vi "testInvalidApplicationRefnum.vi"() -> ()   [LabVIEW 2019, in "AssertionTest.lvlib" / "AssertNotRefnum.lvlib"]
uses:
  AssertNotRefnum.lvlib
  Assertion/Assertion.lvlib
panel:
  out "error out":errorcluster
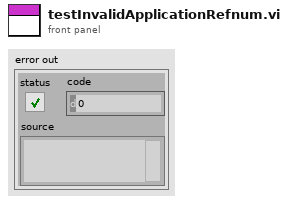
[diagram p1: front panel]
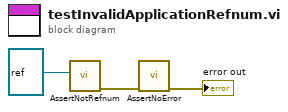
[diagram p0: block diagram]
diagram:
  n1 = call "AssertNotRefnum.vi"("Refnum"=refnum<vi> refnum ("App Refnum")) -> ("error out"=w3:errorcluster)  [unwired: 10 in]
  n2 = call "AssertNoError.vi"("error in (no error)"=w3) -> ("error out"=→"error out":errorcluster)  [unwired: 10 in]
